vi "Write context.vi"(8 "error in (no error)":errorcluster, 10 "zeromq.lvlib:ZeroMQ Context":refnum<class "zmq_context.lvclass">, 11 "Detector in":refnum<class "Detector.lvclass">) -> (0 "error out":errorcluster, 3 "Detector out":refnum<class "Detector.lvclass">)   [LabVIEW 2020, in "Detector.lvclass"]
uses:
  Detector.lvclass
  <vilib>/addons/zeromq/zmq_context.lvclass
  Detector.lvclass/Detector.ctl
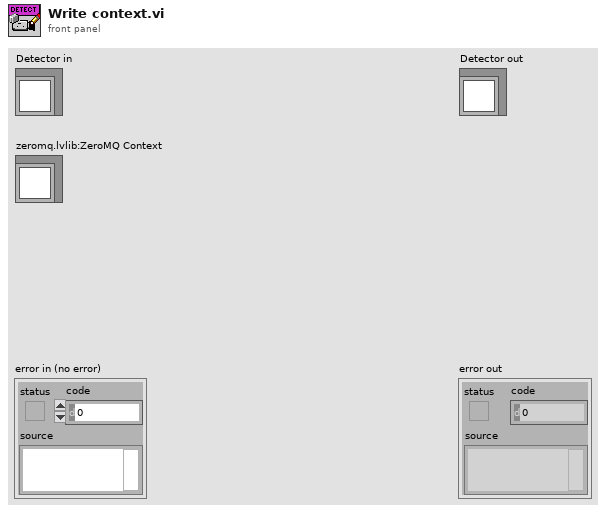
[diagram p1: front panel]
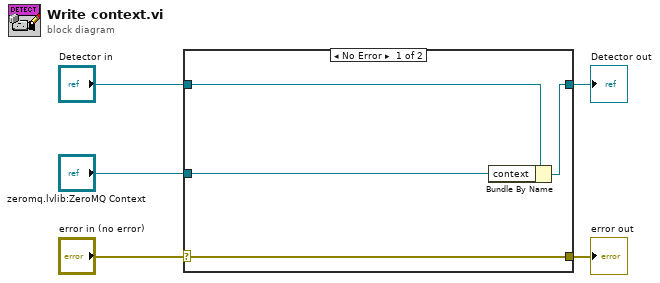
[diagram p0: block diagram]
diagram:
  n1 = case shown="No Error" "error in (no error)" {
    selector: "error in (no error)" -> [w9 w10]
    tunnel: [w9 w10] -> w4
    tunnel: [w7 w11] -> w2
    tunnel: "Detector in" -> [w8 w11]
    tunnel: "zeromq.lvlib:ZeroMQ Context" -> [w6 _]
    frame No Error {
      n2 = Bundle By Name(cluster=w8, "context"=w6) -> (w7:refnum<class "Detector.lvclass">)
    }
    frame Error {
    }
  }
  "error out" <- w4
  "Detector out" <- w2
